vi "MRC Init String.vi"(8 "error in (no error)":errorcluster, 10 "utf8String":string) -> (0 "error out":errorcluster, 2 "str":string, 3 "mrcString out":cluster{"str":u64, "len":i64})   [LabVIEW 2026, in "MrcLib.lvlib"]
doc: "void MRC_CALLCONV MRC_InitString(struct MRC_String* mrcString, const char* utf8String);"
uses:
  MrcLib.lvlib
  MrcLib.dll
  <vilib>/Utility/importsl/GetValueByPointer/GetValueByPointer.xnode
  <vilib>/Utility/importsl/GetValueByPointer/datatype.ctl
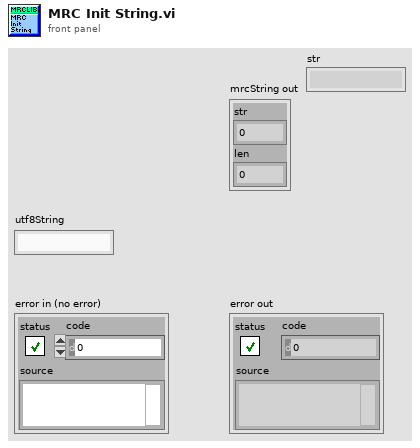
[diagram p1: front panel]
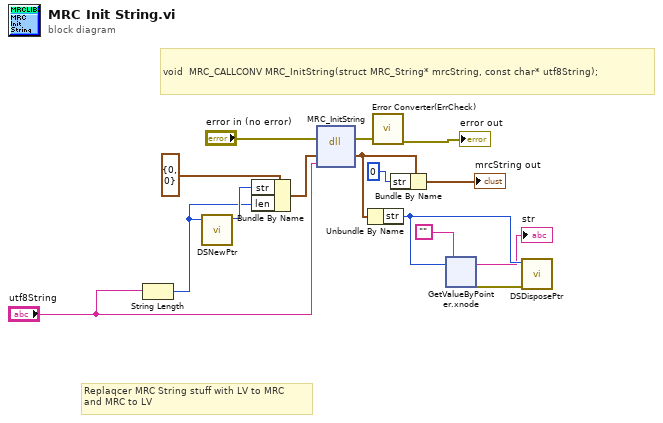
[diagram p0: block diagram]
diagram:
  # "Replaqcer MRC String stuff with LV to MRC\nand MRC to LV"
  # "void  MRC_CALLCONV MRC_InitString(struct MRC_String* mrcString, const char* utf8String);"
  n1 = String Length(string="utf8String") -> (length=w1:i32)
  n2 = call <vilib>:"DSNewPtr.vi"("Size"=w1) -> ("Pointer"=w14:u64)  [unwired: 9 in, 1 out]
  n3 = Bundle By Name(cluster=cluster{"str":u64, "len":i64} {"str"=0, "len"=0} ("mrcString"), "str"=w14, "len"=w1) -> (w13:cluster{"str":u64, "len":i64})
  n4 = dll-call lib="MrcLib.*" fn="MRC_InitString"(error in="error in (no error)", "mrcString"=w13, "utf8String"="utf8String") -> (error out=w4:errorcluster, "mrcString"=w8:cluster{"str":u64, "len":i64})  [unwired: 4 in, 1 out]
  n5 = Unbundle By Name(w8) -> ("str"=w11:u64)
  n6 = call <vilib>:"Error Converter(ErrCheck).vi"("error in (no error)"=w4) -> ("error out"=→"error out":errorcluster)  [unwired: 10 in]
  n7 = Bundle By Name(cluster=w8, "str"=u64 0) -> (→"mrcString out":cluster{"str":u64, "len":i64})
  n8 = xnode "GetValueByPointer.xnode"("Pointer"=w11, "InputType"="") -> ("Output"=→"str":string, "ErrorOut"=w12:errorcluster)  [unwired: 2 in]
  n9 = call <vilib>:"DSDisposePtr.vi"("error in (no error)"=w12, "Pointer"=w11) -> ()  [unwired: 9 in, 1 out]
